vi "Cal Date Valid.vi"(11 "PrevCalDate":i32) -> (1 "Cal Valid?":bool, 3 "Calibration Due Date":string)   [LabVIEW 2019]
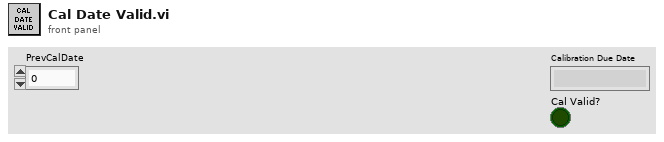
[diagram p1: front panel]
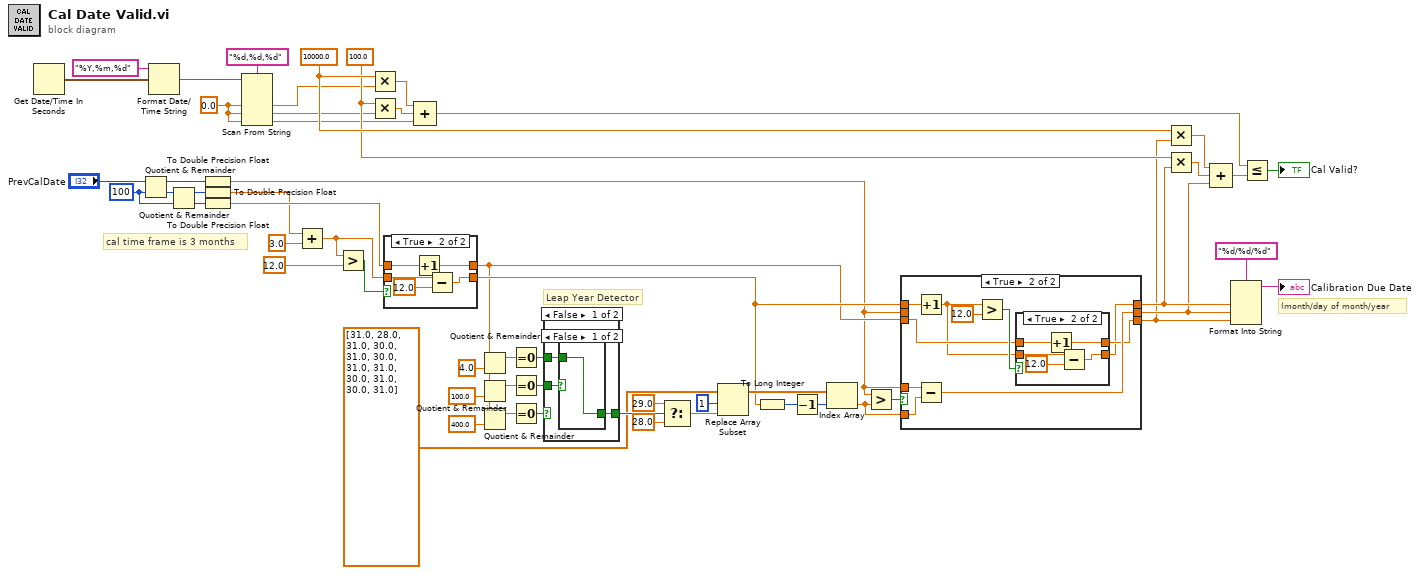
[diagram p0: block diagram]
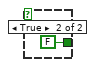
[diagram p4: hidden frame]
diagram:
  w8 = 100 ("y")
  w39 = 0.0 ("x")
  w49 = 10000.0 ("x")
  w48 = 100.0 ("x")
  # "Leap Year Detector"
  # "(month/day of month/year"
  # "cal time frame is 3 months"
  n1 = Get Date/Time In Seconds() -> (seconds since 1Jan1904=w14:timestamp)
  n2 = Quotient & Remainder(x="PrevCalDate", y=w8) -> (x-y*floor(x/y)=w5:i32, floor(x/y)=w7:i32)
  n3 = Format Date/Time String(time format string (%c)="%Y,%m,%d", seconds (now)=w14) -> (date/time string=w12:string)  [unwired: 1 in]
  n4 = Quotient & Remainder(x=w7, y=w8) -> (x-y*floor(x/y)=w4:i32, floor(x/y)=w6:i32)
  n5 = To Double Precision Float(number=w5) -> (double precision float=w1:dbl)
  n6 = To Double Precision Float(number=w4) -> (double precision float=w2:dbl)
  n7 = To Double Precision Float(number=w6) -> (double precision float=w3:dbl)
  n8 = Scan From String(format string="%d,%d,%d", input string=w12, default 1=w39, default 2=w39, default 3=w39) -> (output 1=w43:dbl, output 2=w42:dbl, output 3=w41:dbl)  [unwired: 2 in, 3 out]
  n9 = Add(x=w2, y=3.0) -> (x+y=w56:dbl)
  n10 = Greater?(x=w56, y=12.0) -> (0:w55:bool)
  n11 = Multiply(x=w49, y=w43) -> (x*y=w44:dbl)
  n12 = Multiply(x=w48, y=w42) -> (x*y=w45:dbl)
  n13 = case shown="True" w55 {
    tunnel: w56 -> [w58 w63]
    tunnel: w3 -> [w59 w61]
    tunnel: [w59 w60] -> w15
    tunnel: [w58 w62] -> w20
    frame False {
    }
    frame True {
      n14 = Increment(x=w61) -> (x+1=w60:dbl)
      n15 = Subtract(x=w63, y=12.0) -> (x-y=w62:dbl)
    }
  }
  n16 = Compound Arithmetic op=ADD(w44, w45, w41) -> (w51:dbl)
  n17 = Quotient & Remainder(x=w15, y=4.0) -> (x-y*floor(x/y)=w33:dbl)  [unwired: 1 out]
  n18 = Quotient & Remainder(x=w15, y=100.0) -> (x-y*floor(x/y)=w32:dbl)  [unwired: 1 out]
  n19 = Quotient & Remainder(x=w15, y=400.0) -> (x-y*floor(x/y)=w34:dbl)  [unwired: 1 out]
  n20 = Equal To 0?(x=w33) -> (x = 0?=w29:bool)
  n21 = Equal To 0?(x=w32) -> (x = 0?=w30:bool)
  n22 = Equal To 0?(x=w34) -> (x = 0?=w31:bool)
  n23 = case shown="False" w31 {
    selector: w31 -> [_ w70]
    tunnel: [w66 w70] -> w28
    tunnel: w30 -> [w67 _]
    tunnel: w29 -> [w65 _]
    frame False {
      n24 = case shown="False" w67 {
        tunnel: [w68 FALSE] -> w66
        tunnel: w65 -> [w68 _]
        frame False {
        }
        frame True {
        }
      }
    }
    frame True {
    }
  }
  n25 = Select(t=29.0, s=w28, f=28.0) -> (s? t:f=w27:dbl)
  n26 = Replace Array Subset(array=dbl[] [31.0, 28.0, 31.0, 30.0, 31.0, 30.0, 31.0, 31.0, 30.0, 31.0, 30.0, 31.0], new element=w27, index=1) -> (w22:dbl[])
  n27 = To Long Integer(number=w20) -> (32bit integer=w11:i32)
  n28 = Decrement(x=w11) -> (x-1=w10:i32)
  n29 = Index Array(array=w22, index=w10) -> (element=w19:dbl)
  n30 = Greater?(x=w1, y=w19) -> (0:w21:bool)
  n31 = case shown="True" w21 {
    tunnel: w15 -> [w71 w77]
    tunnel: w20 -> [w73 w78]
    tunnel: w1 -> [w72 _]
    tunnel: [w73 w75] -> w18
    tunnel: [w72 w81] -> w17
    tunnel: [w71 w76] -> w16
    tunnel: w1 -> [_ w83]
    tunnel: w19 -> [_ w82]
    frame False {
    }
    frame True {
      n32 = Increment(x=w78) -> (x+1=w74:dbl)
      n33 = Subtract(x=w83, y=w82) -> (x-y=w81:dbl)
      n34 = Greater?(x=w74, y=12.0) -> (0:w79:bool)
      n35 = case shown="True" w79 {
        tunnel: w74 -> [w84 w89]
        tunnel: w77 -> [w85 w87]
        tunnel: [w85 w86] -> w76
        tunnel: [w84 w88] -> w75
        frame False {
        }
        frame True {
          n36 = Increment(x=w87) -> (x+1=w86:dbl)
          n37 = Subtract(x=w89, y=12.0) -> (x-y=w88:dbl)
        }
      }
    }
  }
  n38 = Multiply(x=w49, y=w16) -> (x*y=w47:dbl)
  n39 = Multiply(x=w48, y=w18) -> (x*y=w46:dbl)
  n40 = Compound Arithmetic op=ADD(w47, w46, w17) -> (w52:dbl)
  n41 = Format Into String(format string="%d/%d/%d", w18, w17, w16) -> (resulting string=→"Calibration Due Date":string)  [unwired: 2 in, 1 out]
  n42 = Less Or Equal?(x=w51, y=w52) -> (x <= y?=→"Cal Valid?":bool)
